vi "read_attributes.vi"(8 "error in (no error)":errorcluster, 11 "StackingClassifier in":refnum<class "StackingClassifier.lvclass">) -> (0 "error out":errorcluster, 2 "attributes":T1, 3 "StackingClassifier out":refnum<class "StackingClassifier.lvclass">)   [LabVIEW 2020, in "StackingClassifier.lvclass"]
uses:
  StackingClassifier.lvclass
  Controls/stacking_classifier_attributes.ctl
  StackingClassifier.lvclass/StackingClassifier.ctl
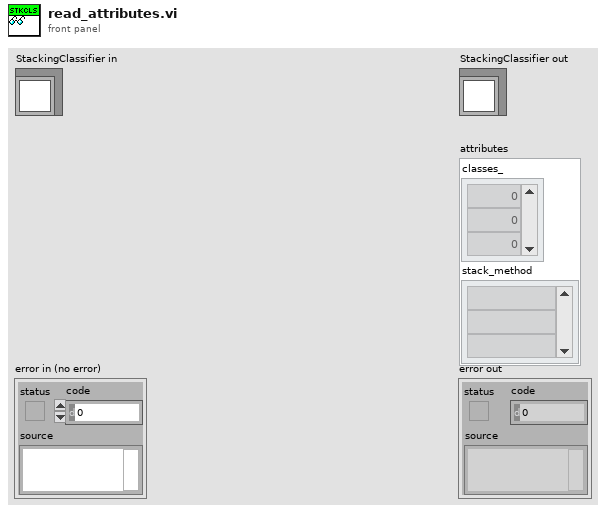
[diagram p1: front panel]
types:
  T1 = typedef "stacking_classifier_attributes.ctl" = cluster{"classes_":dbl[], "stack_method":string[]}
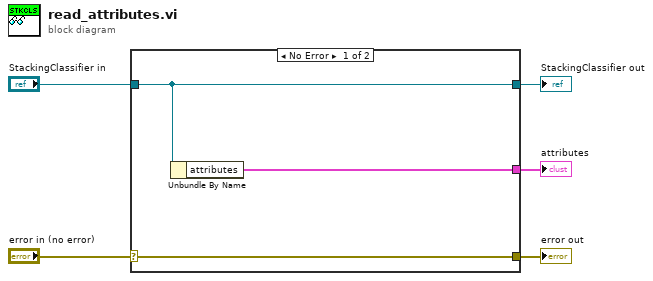
[diagram p0: block diagram]
diagram:
  n1 = case shown="No Error" "error in (no error)" {
    selector: "error in (no error)" -> [w8 w9]
    tunnel: [w8 w9] -> w4
    tunnel: [w7 w10] -> w2
    tunnel: "StackingClassifier in" -> [w7 w10]
    tunnel: [w6 _] -> w1
    frame No Error {
      n2 = Unbundle By Name(w7) -> ("attributes"=w6:T1)
    }
    frame Error {
    }
  }
  "error out" <- w4
  "StackingClassifier out" <- w2
  "attributes" <- w1
